vi "CRYCalc Res Individuall yield.vi"(7 "Step Setup VI No":i32, 8 "Statistic Run Number":i32, 11 "Results in":T2 {"Margin" format="%.2f"}) -> (3 "Individuall Yield Out":T1[](array[typedef]) {"Z data" items=["dB", "Lin"]; "X data" items=["dB", "Lin"]; "Y data" items=["dB", "Lin"]; "Z dB ref" format="%.1f"; "Z axis" items=["Log", "Lin"]; "X dB ref" format="%.1f"; "X axis" items=["Log", "Lin"]; "Y axis" items=["Log", "Lin"]; "Y dB ref" format="%.1f"; "Curve"."z" format="%.2f"; "Curve"."y" format="%.2f"; "Curve"."x" format="%.2f"})   [LabVIEW 2013]
uses:
  Typedef Control/CRYResult Cluster Array.ctl
  Typedef Control/CRYResult Cluster.ctl
  Typedef Control/CRYData Cluster.ctl
  CRYStatistics Global.vi
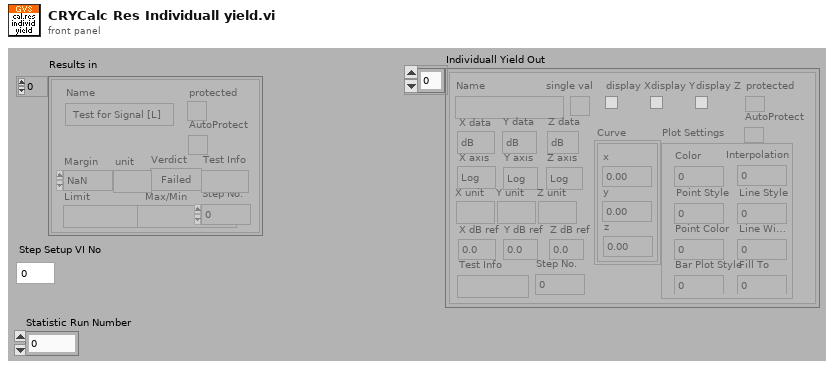
[diagram p1: front panel]
types:
  T1 = typedef "CRYData Cluster.ctl" = cluster{"Name":string, "Curve":cluster{"x":dbl, "y":dbl, "z":dbl}[], "X data":u16, "Y data":u16, "Z data":u16, "X axis":u16, "Y axis":u16, "Z axis":u16, "X unit":string, "Y unit":string, "Z unit":string, "X dB ref":dbl, "Y dB ref":dbl, "Z dB ref":dbl, "single val":bool, "protected":bool, "display X":bool, "display Y":bool, "display Z":bool, "Test Info":string, "Step No.":i32, "Plot Settings":cluster{"Color":u32, "Interpolation":u8, "Point Style":u8, "Line Style":u8, "Point Color":u32, "Line Width":u8, "Bar Plot Style":u8, "Fill To":i16}, "AutoProtect":bool}
  T2 = typedef "CRYResult Cluster Array.ctl" = T3[]
  T3 = typedef "CRYResult Cluster.ctl" = cluster{"Name":string, "Margin":dbl, "unit":string, "Verdict":bool, "Limit":string, "Max/Min":string, "protected":bool, "Step No.":i32, "Test Info":string, "AutoProtect":bool}
  T4 = enum32{"English", "Chinese", "Korean", "Japanese", "Russian", "Chinese traditional"}
  T5 = typedef "CRYData Cluster Array.ctl" = T1[]
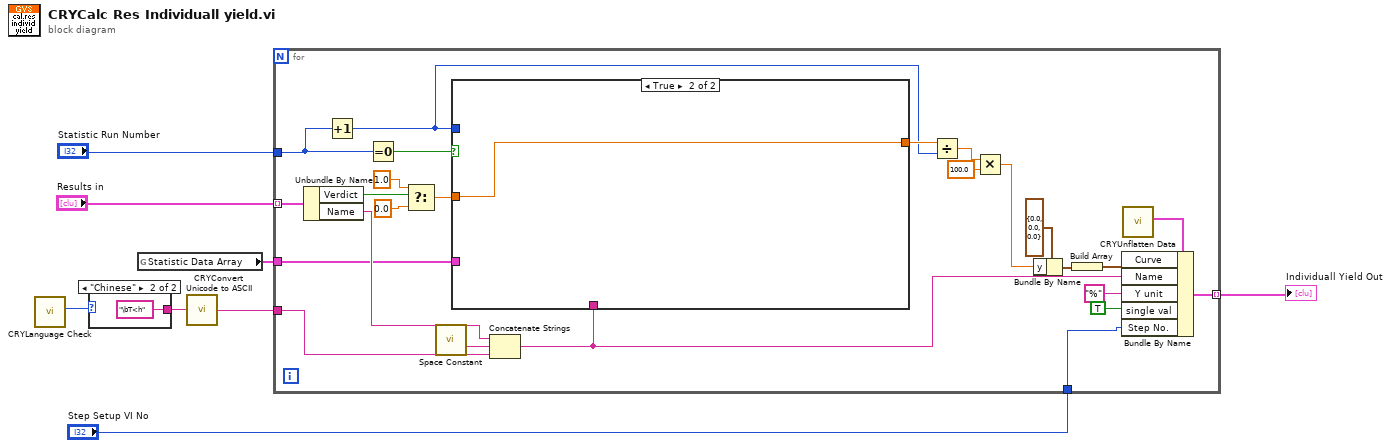
[diagram p0: block diagram]
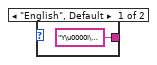
[diagram p2: hidden frame]
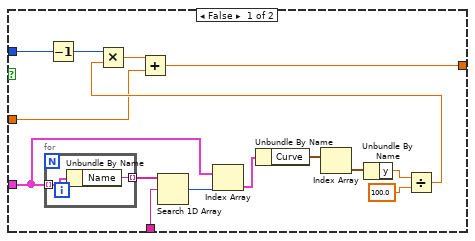
[diagram p3: hidden frame]
diagram:
  n1 = call "CRYLanguage Check.vi"() -> ("Language"=w3:T4)  [unwired: 10 in, 1 out]
  n2 = case shown="\"Chinese\"" w3 {
    tunnel: ["Y\u0000i\u0000e\u0000l\u0000d\u0000" ("format string") "\bT<h" ("format string")] -> w2
    frame "English", Default {
    }
    frame "Chinese" {
    }
  }
  n3 = global read "CRYStatistics Global.vi" "Statistic Data Array"() -> (w6:T5)
  n4 = call "CRYConvert Unicode to ASCII.vi"("Unicode"=w2) -> ("ASCII"=w1:string)  [unwired: 4 in]
  n5 = for {
    tunnel: "Results in" -> [w24] mode=indexing
    tunnel: [w25] -> w7 mode=indexing
    tunnel: w6 -> [w21]
    tunnel: "Statistic Run Number" -> [w15]
    tunnel: "Step Setup VI No" -> [w12]
    tunnel: w1 -> [w11]
    n6 = Unbundle By Name(w24) -> ("Verdict"=w18:bool, "Name"=w23:string)
    n7 = Increment(x=w15) -> (x+1=w13:i32)
    n8 = Equal To 0?(x=w15) -> (x = 0?=w14:bool)
    n9 = Select(t=1.0, s=w18, f=0.0) -> (s? t:f=w17:dbl)
    n10 = call <vilib>:"Space Constant.vi"() -> ("String"=w26:string)
    n11 = Concatenate Strings(w23, w26, w11) -> (w22:string)
    n12 = case shown="True" w14 {
      tunnel: w22 -> [w49 _]
      tunnel: w21 -> [w47 _]
      tunnel: w17 -> [w37 w53]
      tunnel: w13 -> [w40 _]
      tunnel: [w36 w53] -> w16
      frame False {
        n13 = for {
          tunnel: w47 -> [w52] mode=indexing
          tunnel: [w51] -> w50 mode=indexing
          n14 = Unbundle By Name(w52) -> ("Name"=w51:string)
        }
        n15 = Decrement(x=w40) -> (x-1=w39:i32)
        n16 = Search 1D Array(1D array=w50, element=w49) -> (index of element=w48:i32)  [unwired: 1 in]
        n17 = Index Array(array=w47, index=w48) -> (element=w46:T1)
        n18 = Unbundle By Name(w46) -> ("Curve"=w45:cluster{"x":dbl, "y":dbl, "z":dbl}[])
        n19 = Index Array(array=w45) -> (element=w44:cluster{"x":dbl, "y":dbl, "z":dbl})  [unwired: 1 in]
        n20 = Unbundle By Name(w44) -> ("y"=w43:dbl)
        n21 = Divide(x=w43, y=100.0) -> (x/y=w41:dbl)
        n22 = Multiply(x=w39, y=w41) -> (x*y=w38:dbl)
        n23 = Add(x=w38, y=w37) -> (x+y=w36:dbl)
      }
      frame True {
      }
    }
    n24 = Divide(x=w16, y=w13) -> (x/y=w28:dbl)
    n25 = Multiply(x=w28, y=100.0) -> (x*y=w30:dbl)
    n26 = Bundle By Name(cluster=cluster{"x":dbl, "y":dbl, "z":dbl} {"x"=0.0, "y"=0.0, "z"=0.0}, "y"=w30) -> (w35:cluster{"x":dbl, "y":dbl, "z":dbl})
    n27 = Build Array(w35) -> (w31:cluster{"x":dbl, "y":dbl, "z":dbl}[])
    n28 = call "CRYUnflatten Data.vi"() -> ("Datum"=w29:T1)  [unwired: 9 in, 2 out]
    n29 = Bundle By Name(cluster=w29, "Curve"=w31, "Name"=w22, "Y unit"="%", "single val"=TRUE, "Step No."=w12) -> (w25:T1)
  }
  "Individuall Yield Out" <- w7
